vi "Is_TestDataInSpec-单值.vi"(1 "量测规格":T1 {"上限" format="%#.4g"; "下限" format="%#.4g"}, 2 "相机量测结果":dbl) -> (0 "在规格内":bool)   [LabVIEW 2014]
uses:
  Controls/TestThreshold.ctl
panel:
  # "~"
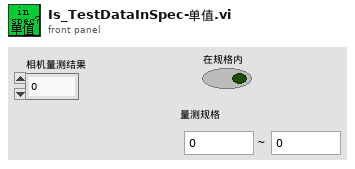
[diagram p1: front panel]
types:
  T1 = typedef "TestThreshold.ctl" = cluster{"下限":dbl, "上限":dbl}
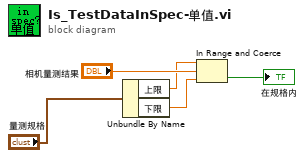
[diagram p0: block diagram]
diagram:
  n1 = Unbundle By Name("量测规格") -> ("上限"=w2:dbl, "下限"=w3:dbl)
  n2 = In Range and Coerce(upper limit=w2, x="相机量测结果", lower limit=w3) -> (In Range?=→"在规格内":bool)  [unwired: 1 out]
